vi "Write TDMS File.vi"(8 "error in (no error)":errorcluster, 10 "Data":dbl[](array[numeric]), 11 "Path":path) -> (0 "error out":errorcluster)   [LabVIEW 2015]
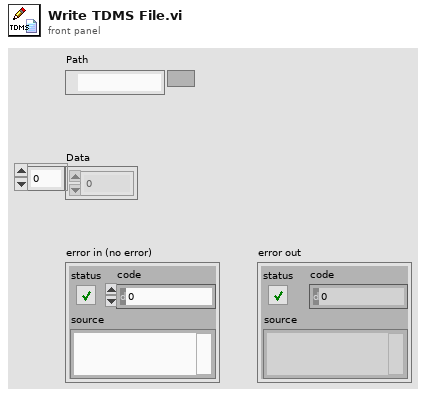
[diagram p1: front panel]
types:
  T1 = enum16{"open", "open or create", "create or replace", "create", "open (read-only)"}
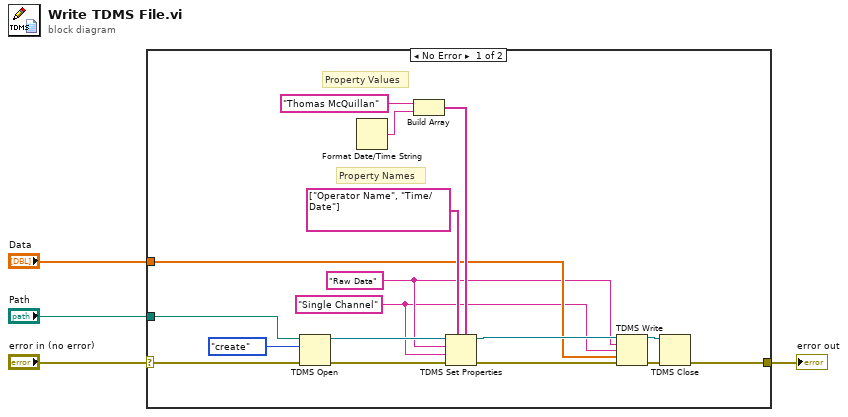
[diagram p0: block diagram]
diagram:
  n1 = case shown="No Error" "error in (no error)" {
    selector: "error in (no error)" -> [w13 w22]
    tunnel: [w11 w22] -> w3
    tunnel: "Data" -> [w7 _]
    tunnel: "Path" -> [w12 _]
    frame No Error {
      w5 = "Single Channel" ("group name")
      w6 = "Raw Data" ("group name")
      # "Property Values"
      # "Property Names"
      n2 = TDMS Open(8:w13, 10:T1."create" ("operation (0:open)"), 11:w12) -> (0:w18:errorcluster, 3:w19:refnum<k34>)  [unwired: 4 in]
      n3 = Format Date/Time String() -> (date/time string=w20:string)  [unwired: 3 in]
      n4 = Build Array("Thomas McQuillan", w20) -> (w8:string[])
      n5 = TDMS Set Properties(5:w8, 7:string[] ["Operator Name", "Time/Date"], 8:w18, 9:w5, 10:w6, 11:w19) -> (0:w16:errorcluster, 3:w17:refnum<k34>)  [unwired: 2 out]
      n6 = TDMS Write(0:w17, 5:w6, 7:w5, 9:w7, 11:w16) -> (4:w15:refnum<k34>, 15:w14:errorcluster)  [unwired: 1 in, 2 out]
      n7 = TDMS Close(8:w14, 11:w15) -> (0:w11:errorcluster)  [unwired: 1 out]
    }
    frame Error {
    }
  }
  "error out" <- w3
